vi "Save Test Executive.vi"(4 "File Name":string, 5 "New GUIDs":bool, 6 "Folder":path, 7 "Persistence in":refnum<class "IPersist.lvclass">, 8 "error in (no error)":errorcluster, 11 "Test Executive Ref":refnum<data-value>) -> (0 "error out":errorcluster, 3 "Test Executive Ref out":refnum<data-value>)   [LabVIEW 2017, in "Test Executive.lvlib" / "TestExecutive Ref.lvclass"]
uses:
  <vilib>/gpm_packages/@cs/test-executive/Source/Test Executive/TestExecutive Ref/TestExecutive Ref.lvclass
  <vilib>/gpm_packages/@cs/test-executive/Source/Test Executive/ITestExecutive/ITest Executive.lvclass
  <vilib>/gpm_packages/@cs/persistence/source/IPersist/IPersist.lvclass
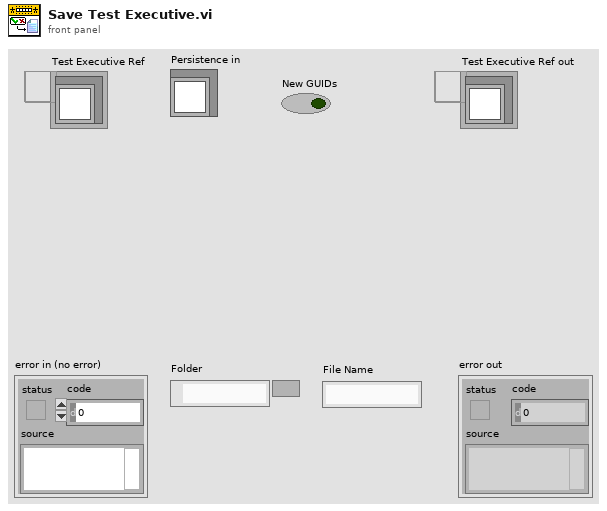
[diagram p1: front panel]
types:
  T1 = enum16{"open", "replace", "create", "open or create", "replace or create", "replace or create with confirmation"}
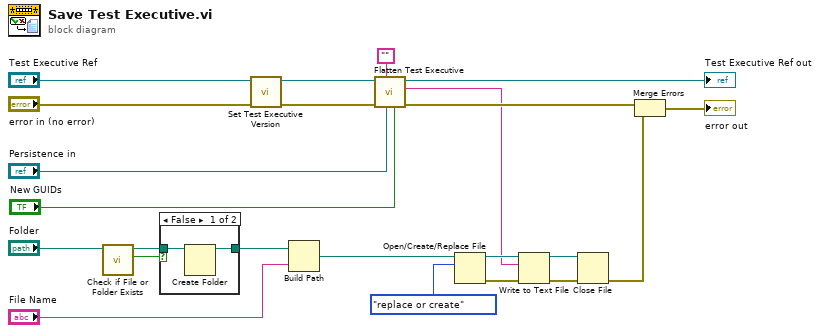
[diagram p0: block diagram]
diagram:
  n1 = call <vilib>:"Check if File or Folder Exists.vi"("path"="Folder") -> ("file or folder exists?"=w11:bool, "dup path"=w12:path)  [unwired: 8 in, 1 out]
  n2 = case shown="False" w11 {
    tunnel: w12 -> [w25 w26]
    tunnel: [w24 w26] -> w13
    frame False {
      n3 = Create Folder(path (use dialog)=w25) -> (created path=w24:path)  [unwired: 2 in, 2 out]
    }
    frame True {
    }
  }
  n4 = call <vilib>:"Set Test Executive Version.vi"("error in (no error)"="error in (no error)", "Test Executive Ref"="Test Executive Ref") -> ("error out"=w2:errorcluster, "Test Executive Ref out"=w4:refnum<data-value>)  [unwired: 8 in]
  n5 = Build Path(base path=w13, name or relative path="File Name") -> (appended path=w6:path)
  n6 = call <vilib>:"Flatten Test Executive.vi"("New GUIDs"="New GUIDs", "Persistence in"="Persistence in", "Root ID"="", "error in (no error)"=w2, "Test Executive Ref"=w4) -> ("error out"=w21:errorcluster, "Flattened Test Executive"=w8:string, "Test Executive Ref out"=→"Test Executive Ref out":refnum<data-value>)  [unwired: 4 in]
  n7 = Open/Create/Replace File(file path (use dialog)=w6, operation (0:open)=T1."replace or create") -> (refnum out=w15:refnum<file>, error out=w17:errorcluster)  [unwired: 4 in, 1 out]
  n8 = Write to Text File(file (use dialog)=w15, text=w8, error in=w17) -> (refnum out=w16:refnum<file>, error out=w18:errorcluster)  [unwired: 1 in, 1 out]
  n9 = Close File(refnum=w16, error in=w18) -> (error out=w7:errorcluster)  [unwired: 1 out]
  n10 = Merge Errors(w21, w7) -> (→"error out":errorcluster)
